vi "Wait and Read Return (SubVI).vi"(8 "Fehler (Eingang, kein Fehler)":errorcluster, 11 "VISA-Referenz (Eingang)":refnum<visa-resource-name>) -> (0 "Fehler (Ausgang)":errorcluster, 2 "Antwort":string, 3 "VISA-Referenz (Ausgang)":refnum<visa-resource-name>)   [LabVIEW 2017]
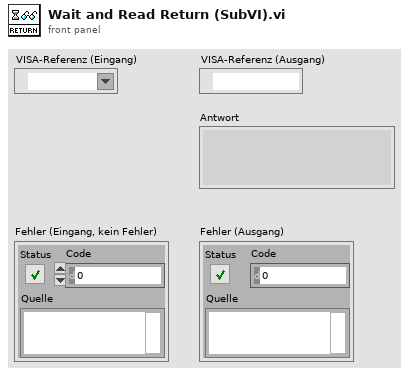
[diagram p1: front panel]
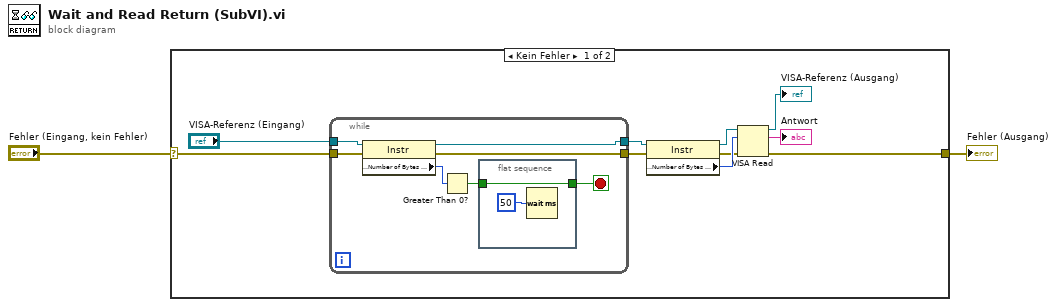
[diagram p0: block diagram]
diagram:
  n1 = case shown="Kein Fehler" "Fehler (Eingang, kein Fehler)" {
    selector: "Fehler (Eingang, kein Fehler)" -> [w8 w22]
    tunnel: [w11 w22] -> w2
    frame No Error {
      n2 = while {
        tunnel: "VISA-Referenz (Eingang)" -> [w19]
        tunnel: w8 -> [w18]
        tunnel: [w17] -> w7
        tunnel: [w15] -> w4
        stop <- w14 stop-if-true
        n3 = property class="Instr"(reference=w19, error in=w18) -> (reference out=w17:refnum<visa-resource-name>, error out=w15:errorcluster, "Serial Settings:Number of Bytes at Serial Port"=w16:u32)
        n4 = Greater Than 0?(x=w16) -> (x > 0?=w13:bool)
        n5 = flat-sequence {
          tunnel: [w20] -> w14
          tunnel: w13 -> [w20]
          frame #0 {
            n6 = Wait (ms)(milliseconds to wait=u32 50 ("Zu wartende ms")) -> ()  [unwired: 1 out]
          }
        }
      }
      n7 = property class="Instr"(reference=w7, error in=w4) -> (reference out=w5:refnum<visa-resource-name>, error out=w3:errorcluster, "Serial Settings:Number of Bytes at Serial Port"=w6:u32)
      n8 = VISA Read(VISA resource name=w5, byte count=w6, error in (no error)=w3) -> (VISA resource name out=→"VISA-Referenz (Ausgang)":refnum<visa-resource-name>, read buffer=→"Antwort":string, error out=w11:errorcluster)  [unwired: 1 out]
    }
    frame Error {
    }
  }
  "Fehler (Ausgang)" <- w2
